vi "qERR.vi"(0 "System no.":i32=1 min=1 max=4 step=1, 5 "error in":errorcluster) -> (14 "Controller error":bool, 19 "error out":errorcluster)   [LabVIEW 2026]
doc: "GCS 3.0\n=====\n\nERR? (Get Error)\n\nDescription \nQueries the error code that is currently stored in the GCS interpreter of the communication \ninterface used.\n\nFormat\nERR?\n\nArguments\nnone\n\nResponse\nThe error code that is currently stored in the GCS interpreter of the communication interface \nused.\nIf no error code has been stored in the GCS interpreter of the communication interface used \nsince ERR? was last sent, the next ERR? on the same interface will return the value 0.\n\nExample\n>>cst?\n>>err?\n<<49155 - (error 49155 - \"Unknown command\")\n>>err?\n<<0 - (error 0 - \"No error\")\n>>log?\n<<#Error Information: <Index> <Timestamp> <Error Code>\n<Error Class> <Container Unit><Function Unit>\n<<1 17375192000000 49155 CMD SYS_1 INTPR_1\n<<2 17628935000000 49217 CMD SYS_1 INTPR_1\n<<3 17780977000000 49155 CMD SYS_1 INTPR_1\n<<#END Error Information\n>>log?\n<<#Error Information: <Index> <Timestamp> <Error Code>\n<Error Class> <Container Unit><Function Unit>\n<<1 17375192000000 49155 CMD SYS_1 INTPR_1\n<<2 17628935000000 49217 CMD SYS_1 INTPR_1\n<<3 17780977000000 49155 CMD SYS_1 INTPR_1\n<<#END Error Information\n\nNotes\nIn GCS 3.0, errors that occur during operation of the controller are recorded and output as \nfollows:\n- After switching on/rebooting the controller, all errors are logged globally and stored \ntemporarily. The contents of the log memory can be queried with the LOG? command. \n- The ERR? command queries the error code that is currently stored in the GCS \ninterpreter of the communication interface used. Only errors of the Command class are \nstored in the GCS interpreters of the controller.\n- The status register of an axis shows whether an error of the Motion class is \npresent for the axis (i.e. a motion error). The status register of an axis can be queried \nwith the STV? command. \n- The status register of the system shows whether there are errors from the \nclasses Command, Critical, Warning and Info. The status register of the system can be \nqueried with the STV? command. \nUser software could, for example, use the bits of the status registers as trigger for querying the \nlog memory.\nThe error code corresponds to the <Error Code> field from the response to the LOG? command.\nFor further information, see \"Error Handling - GCS 3.0\". \n\nUser command level\nUSR\n\n\nGCS 2.0\n=====\n\nReturns error information. Controller error is TRUE if selected system reports an error code which is not 0. See appendix A of the GCS LabVIEW manual for a list of PI error codes and use GCSTranslateError.vi to translate error codes into error descriptions programmatically.\n\nAnalog system: VI does not report any error.\nE-816: This command cannot be issued to a slave."
panel:
  # "ERR? (Get Error)\n\nQueries the error code that is currently stored in the GCS interpreter of the communication interface used."
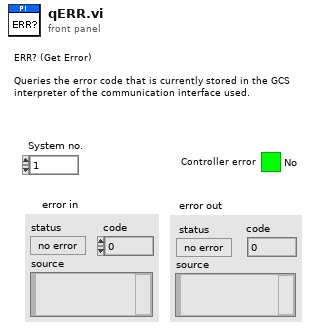
[diagram p1: front panel]
types:
  T1 = enum16{"Disable error check", "Force error check", "Use global settings"}
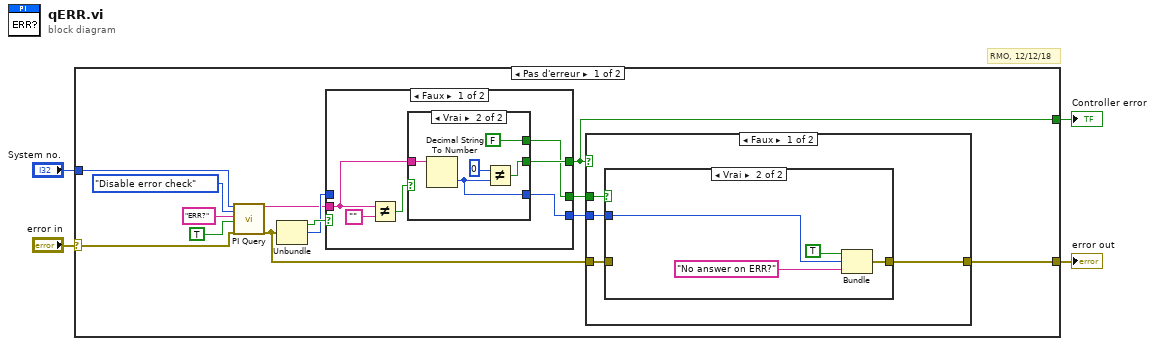
[diagram p0: block diagram]
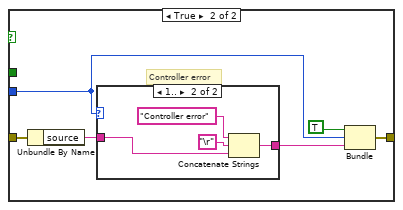
[diagram p3: hidden frame]
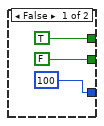
[diagram p5: hidden frame]
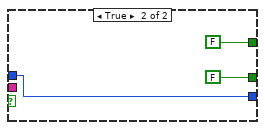
[diagram p6: hidden frame]
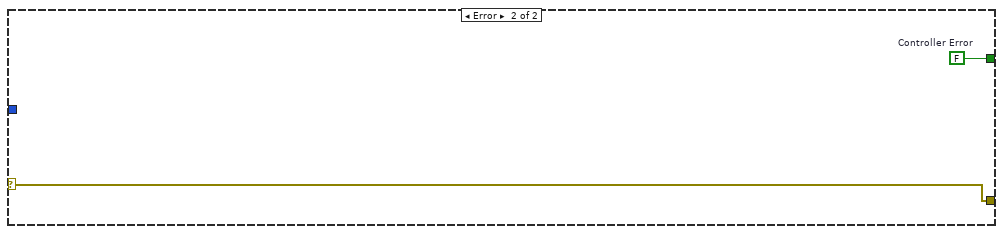
[diagram p7: hidden frame]
diagram:
  # "RMO, 12/12/18"
  n1 = case shown="Pas d'erreur" "error in" {
    selector: "error in" -> [w5 w56]
    tunnel: [w15 w55] -> w4
    tunnel: [w13 w56] -> w3
    tunnel: "System no." -> [w10 _]
    frame No Error {
      n2 = call "PI Query.vi"("System no."=w10, "Error check settings"=T1."Disable error check", "String to send"="ERR?", "Attach termination char.?"=TRUE ("Attach Linefeed?"), "error in"=w5) -> ("String read"=w8:string, "error out"=w7:errorcluster)  [unwired: 2 in, 11 out]
      n3 = Unbundle(w7) -> ("status"=w16:bool, "code"=w12:i32)  [unwired: 1 out]
      n4 = case shown="Faux" w16 {
        tunnel: w8 -> [w41 _]
        tunnel: [w43 FALSE ("Controller Error")] -> w15
        tunnel: [w42 w53] -> w14
        tunnel: w12 -> [_ w53]
        tunnel: [w38 FALSE ("Controller Error")] -> w9
        frame False {
          n5 = Not Equal?(x=w41, y="") -> (x != y?=w40:bool)
          n6 = case shown="Vrai" w40 {
            tunnel: [FALSE w51] -> w43
            tunnel: w41 -> [_ w49]
            tunnel: [100 w48] -> w42
            tunnel: [TRUE FALSE] -> w38
            frame False {
            }
            frame True {
              n7 = Decimal String To Number(string=w49) -> (number=w48:i32)  [unwired: 3 out]
              n8 = Not Equal?(x=0, y=w48) -> (x != y?=w51:bool)
            }
          }
        }
        frame True {
        }
      }
      n9 = case shown="Faux" w15 {
        tunnel: w14 -> [w18 w30]
        tunnel: [w20 w32] -> w13
        tunnel: w7 -> [w21 w28]
        tunnel: w9 -> [w19 _]
        frame False {
          n10 = case shown="Vrai" w19 {
            tunnel: w21 -> [w22 _]
            tunnel: [w22 w23] -> w20
            tunnel: w18 -> [_ w25]
            frame False {
            }
            frame True {
              n11 = Bundle("status"=TRUE, "code"=w25, "No answer on ERR?") -> (w23:cluster{"status":bool, "code":i32, string})  [unwired: 1 out]
            }
          }
        }
        frame True {
          # "Controller error"
          n12 = Unbundle By Name(w28) -> ("source"=w27:string)
          n13 = case shown="1.." w30 {
            tunnel: [w33 w37] -> w29
            tunnel: w27 -> [w33 w35]
            frame ..0 {
            }
            frame 1.. {
              n14 = Concatenate Strings("Controller error", "\r" ("Substring"), w35) -> (w37:string)
            }
          }
          n15 = Bundle("status"=TRUE, "code"=w30, "source"=w29) -> (w32:errorcluster)  [unwired: 1 out]
        }
      }
    }
    frame Error {
      w55 = FALSE  # Controller Error
    }
  }
  "Controller error" <- w4
  "error out" <- w3
